vi "Devices Available.vi"(8 "error in (no error)":errorcluster) -> (0 "error out":errorcluster, 1 "Default Device":tag, 2 "DevNames":tag[](array[tag]), 3 "Devices":string[](array[string]), 4 "# devices":i32)   [LabVIEW 2019]
uses:
  <resource>/objmgr/daqmx.rc
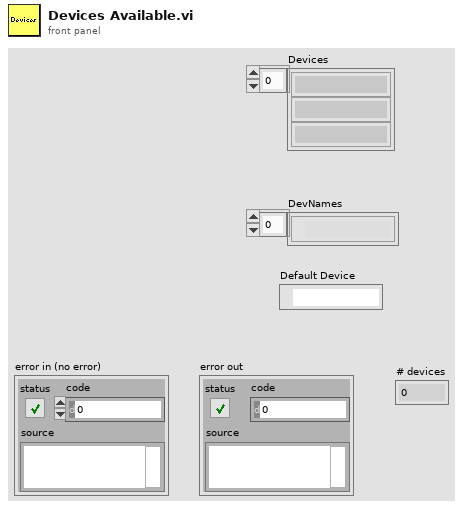
[diagram p1: front panel]
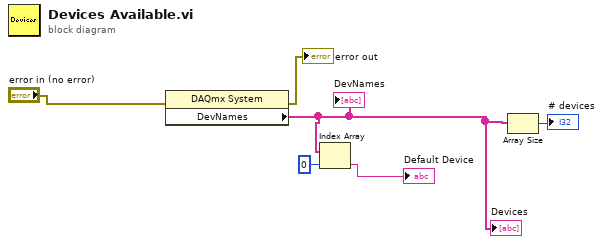
[diagram p0: block diagram]
diagram:
  n1 = property class="DAQmx System"(error in="error in (no error)") -> (error out=→"error out":errorcluster, "DevNames"=w2:tag[])  [unwired: 1 in, 1 out]
  "Devices" <- w2
  "DevNames" <- w2
  n2 = Index Array(array=w2, index=0) -> (element=→"Default Device":tag)
  n3 = Array Size(array=w2) -> (size(s)=→"# devices":i32)
